vi "labjack.vi"() -> ()   [LabVIEW 2013]
panel:
  in  "On/Off":bool
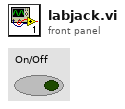
[diagram p1: front panel]
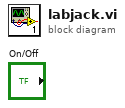
[diagram p0: block diagram]
diagram:
